vi "Boiler room teest 2.vi"() -> ()   [LabVIEW 2023]
uses:
  Heater.vi
  AC.vi
panel:
  out "temp":dbl
  in  "Heater":dbl(knob) min=0.0 max=2.0 step=1.0 scale=0.0..2.0
  in  "stop":bool
  out "Thermometer":dbl(slide) scale=0.0..100.0
  in  "min temp":dbl=20.0
  in  "max temp":dbl=80.0
  in  "Automatic / Manual":bool
  out "AC":bool
  out "Heater":bool
  # "OFF"
  # "AC"
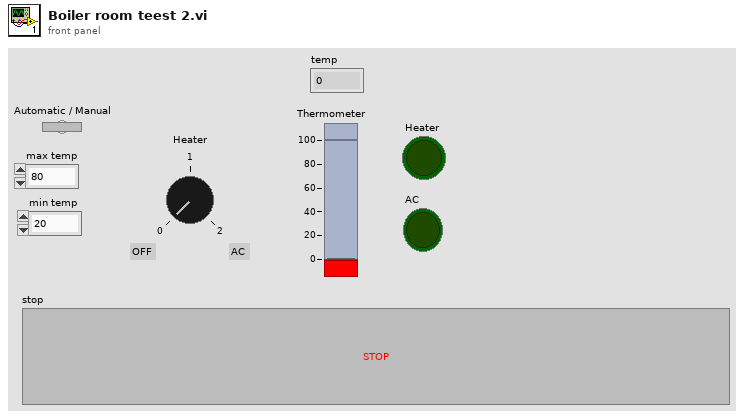
[diagram p1: front panel]
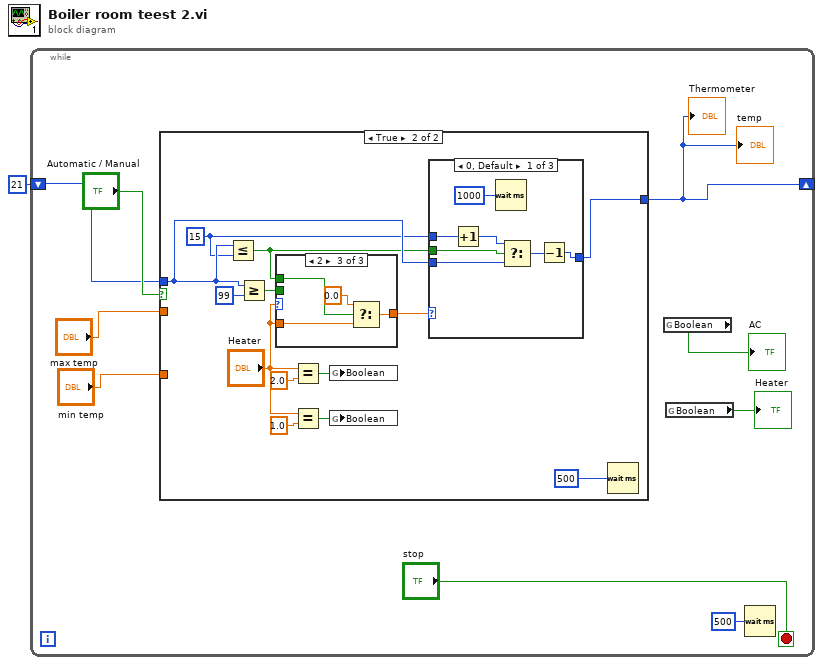
[diagram p0: block diagram]
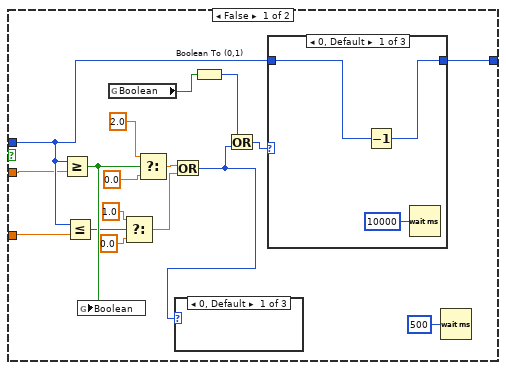
[diagram p2: hidden frame]
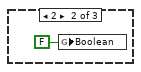
[diagram p3: hidden frame]
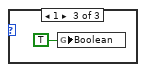
[diagram p4: hidden frame]
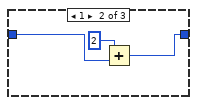
[diagram p5: hidden frame]
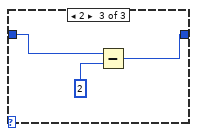
[diagram p6: hidden frame]
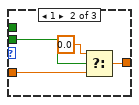
[diagram p8: hidden frame]
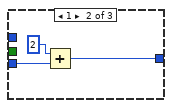
[diagram p9: hidden frame]
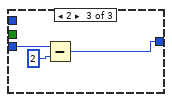
[diagram p10: hidden frame]
diagram:
  n1 = while {
    shift-right: [w5] -> _
    shift-left: 21 -> [w2]
    stop <- "stop" stop-if-true
    n2 = case shown="True" "Automatic / Manual" {
      tunnel: w2 -> [w20 w44]
      tunnel: "max temp" -> [w19 _]
      tunnel: "min temp" -> [w18 _]
      tunnel: [w22 w50] -> w5
      frame False {
        n3 = Greater Or Equal?(x=w20, y=w19) -> (x >= y?=w16:bool)
        n4 = Less Or Equal?(x=w20, y=w18) -> (x <= y?=w15:bool)
        n5 = global write "AC.vi" "Boolean"(w16) -> ()
        n6 = global read "Heater.vi" "Boolean"() -> (w11:bool)
        n7 = Select(t=1.0, s=w15, f=0.0) -> (s? t:f=w17:dbl)
        n8 = Select(t=2.0, s=w16, f=0.0) -> (s? t:f=w23:dbl)
        n9 = Or(x=w23, y=w17) -> (x .or. y?=w14:i32)
        n10 = case shown="0, Default" w14 {
          frame 0, Default {
          }
          frame 2 {
            n11 = global write "Heater.vi" "Boolean"(FALSE ("Boolean")) -> ()
          }
          frame 1 {
            n12 = global write "Heater.vi" "Boolean"(TRUE ("Boolean")) -> ()
          }
        }
        n13 = Boolean To (0,1)(Boolean=w11) -> (0, 1=w12:i16)
        n14 = Or(x=w12, y=w14) -> (x .or. y?=w13:i32)
        n15 = case shown="0, Default" w13 {
          tunnel: w20 -> [w32 w35 w38]
          tunnel: [w31 w33 w37] -> w22
          frame 0, Default {
            n16 = Decrement(x=w32) -> (x-1=w31:i32)
            n17 = Wait (ms)(milliseconds to wait=u32 10000) -> ()  [unwired: 1 out]
          }
          frame 1 {
            n18 = Add(x=2, y=w35) -> (x+y=w33:i32)
          }
          frame 2 {
            n19 = Subtract(x=w38, y=2) -> (x-y=w37:i32)
          }
        }
        n20 = Wait (ms)(milliseconds to wait=u32 500) -> ()  [unwired: 1 out]
      }
      frame True {
        w39 = 15
        n21 = Less Or Equal?(x=w44, y=w39) -> (x <= y?=w40:bool)
        n22 = Greater Or Equal?(x=w44, y=99 ("x")) -> (x >= y?=w41:bool)
        n23 = case shown="2" "Heater" {
          tunnel: "Heater" -> [w52 w53 w58]
          tunnel: [w52 w55 w59] -> w49
          tunnel: w41 -> [_ w56 _]
          tunnel: w40 -> [_ _ w60]
          frame 0, Default {
          }
          frame 1 {
            n24 = Select(t=0.0 ("f"), s=w56, f=w53) -> (s? t:f=w55:dbl)
          }
          frame 2 {
            n25 = Select(t=0.0, s=w60, f=w58) -> (s? t:f=w59:dbl)
          }
        }
        n26 = Equal?(x="Heater", y=2.0) -> (x = y?=w45:bool)
        n27 = Equal?(x="Heater", y=1.0) -> (x = y?=w47:bool)
        n28 = global write "AC.vi" "Boolean"(w45) -> ()
        n29 = global write "Heater.vi" "Boolean"(w47) -> ()
        n30 = case shown="0, Default" w49 {
          tunnel: w44 -> [w64 w70 w73]
          tunnel: [w67 w69 w72] -> w50
          tunnel: w40 -> [w65 _ _]
          tunnel: w39 -> [w62 _ _]
          frame 0, Default {
            n31 = Increment(x=w62) -> (x+1=w61:i32)
            n32 = Wait (ms)(milliseconds to wait=u32 1000) -> ()  [unwired: 1 out]
            n33 = Select(t=w61, s=w65, f=w64) -> (s? t:f=w63:i32)
            n34 = Decrement(x=w63) -> (x-1=w67:i32)
          }
          frame 1 {
            n35 = Add(x=2, y=w70) -> (x+y=w69:i32)
          }
          frame 2 {
            n36 = Subtract(x=w73, y=2) -> (x-y=w72:i32)
          }
        }
        n37 = Wait (ms)(milliseconds to wait=u32 500) -> ()  [unwired: 1 out]
      }
    }
    "Thermometer" <- w5
    "temp" <- w5
    n38 = global read "AC.vi" "Boolean"() -> (→"AC":bool)
    n39 = global read "Heater.vi" "Boolean"() -> (→"Heater":bool)
    n40 = Wait (ms)(milliseconds to wait=u32 500) -> ()  [unwired: 1 out]
  }
